vi "Center_171213.vi"(9 "DiameterOfTheCenter":u16, 10 "Center":enum16{"1", "0"}(ring), 11 "InputBackground":picture) -> (2 "Colors":u32[](array[numeric]), 3 "OutputBackground":picture)   [LabVIEW 2016]
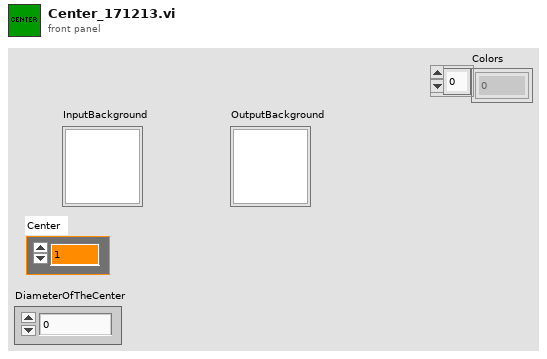
[diagram p1: front panel]
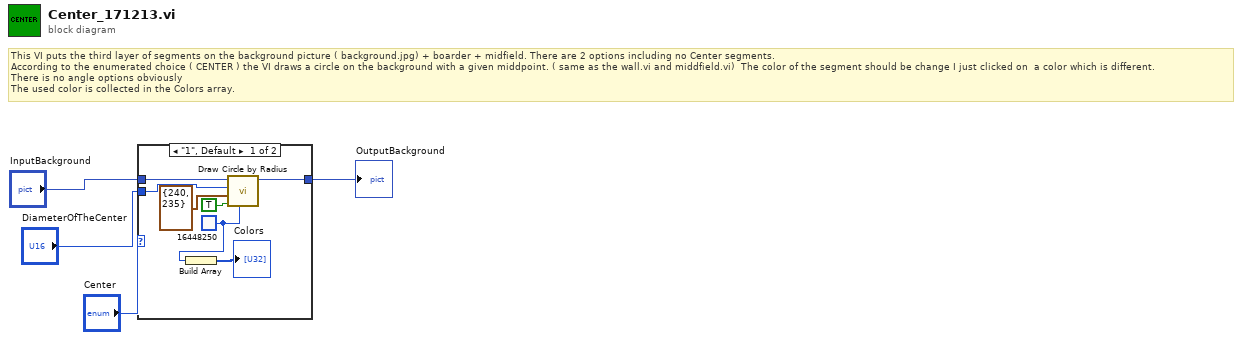
[diagram p0: block diagram]
diagram:
  # "This VI puts the third layer of segments on the background picture ( background.jpg) + boarder + midfield. There are 2 options including no Center segments.\nAccording to the enumerated choice ( CENTER ) the VI draws a circle on the background with a given middpoint. ( same as the wall.vi and middfield.vi)  The color of the segment should be change I just clicked on  a color which is different. \nThere is no angle options obviously\nThe used color is collected in the Colors array."
  n1 = case shown="\"1\", Default" "Center" {
    tunnel: "InputBackground" -> [w8 w12]
    tunnel: [w9 w12] -> w1
    tunnel: "DiameterOfTheCenter" -> [w7 _]
    frame "1", Default {
      w6 = u32 16448250 ("color(black)")
      n2 = Build Array(w6) -> (→"Colors":u32[])
      n3 = call <vilib>:"Draw Circle by Radius.vi"("color(black)"=w6, "fill?(F)"=TRUE, "pixel center"=cluster{"horizontal":i16, "vertical":i16} {"horizontal"=240, "vertical"=235}, "radius"=w7, "picture"=w8) -> ("new picture"=w9:picture)  [unwired: 6 in]
    }
    frame "0" {
    }
  }
  "OutputBackground" <- w1
